vi "ErrorHandler.vi"(8 "error in (no error)":errorcluster, 11 "MessageQueue":refnum<queue>) -> (0 "error out":errorcluster, 3 "MessageQueue":refnum<queue>)   [LabVIEW 2018, in "SensorPlugins.lvlib"]
doc: "This VI places any error that passes through at the front of the queue."
uses:
  SensorPlugins.lvlib
  clMessage.ctl
panel:
  in  "Message (Error)":string="Error"
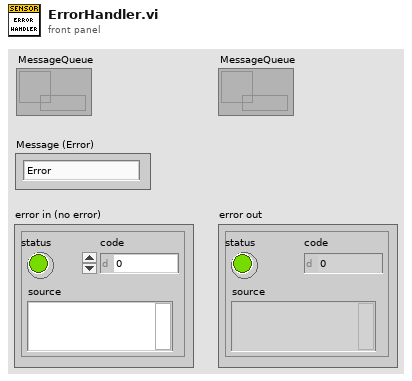
[diagram p1: front panel]
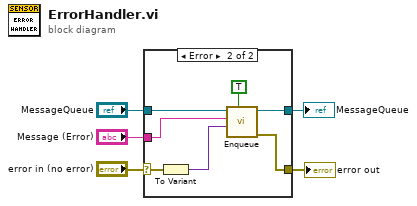
[diagram p0: block diagram]
diagram:
  n1 = case shown="Error" "error in (no error)" {
    selector: "error in (no error)" -> [w6 w13]
    tunnel: [w7 w10] -> w3
    tunnel: "MessageQueue" -> [w7 w14]
    tunnel: "Message (Error)" -> [_ w11]
    tunnel: [w6 w8] -> w1
    frame No Error {
    }
    frame Error {
      n2 = To Variant(anything=w13) -> (Variant=w12:variant)
      n3 = call "Enqueue.vi"("Priority (F)"=TRUE, "Message Data"=w12, "Message"=w11, "MessageQueue"=w14) -> ("error out"=w8:errorcluster, "MessageQueue"=w10:refnum<queue>)  [unwired: 6 in]
    }
  }
  "error out" <- w1
  "MessageQueue" <- w3
